vi "Default Settings.vi"(6 "Assembly Type":string, 8 "error in (no error)":errorcluster, 11 "Sensor Dispense in":refnum<class "Sensor Dispense.lvclass">) -> (0 "error out":errorcluster, 3 "Sensor Dispense out":refnum<class "Sensor Dispense.lvclass">)   [LabVIEW 2021, in "Sensor Dispense.lvclass"]
uses:
  Projects/Sensor Dispense.lvclass
  C:/Users/User/Documents/Jessica_Code/Jessica_code_06052024/Gantry-CMU/UCSB-Gantry-HEP-main/Classes/Routine/Dispense/Dispense.lvclass
  Projects/Sensor Dispense.lvclass/Sensor Dispense.ctl
  Dispense.lvclass/Dispense.ctl
  Write Tip Height.vi
  Dispense.lvclass
panel:
  in  "Dispense Type":u16
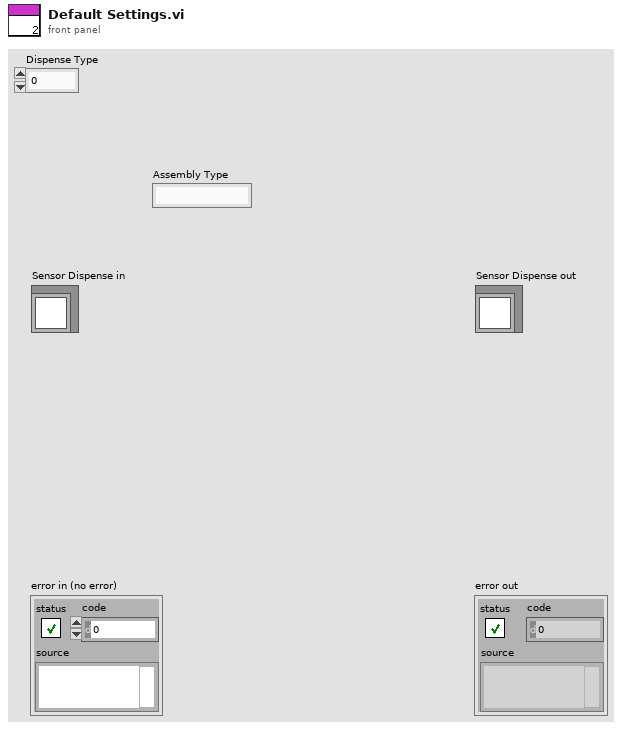
[diagram p1: front panel]
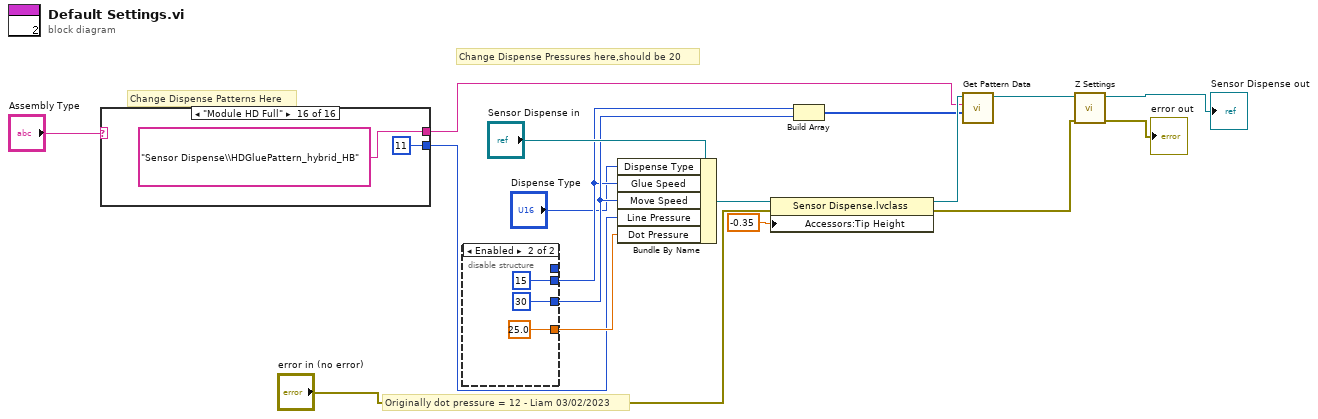
[diagram p0: block diagram]
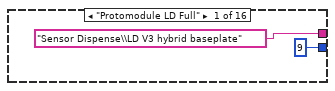
[diagram p2: hidden frame]
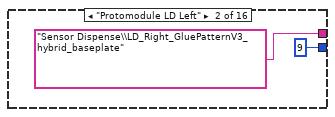
[diagram p3: hidden frame]
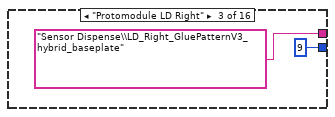
[diagram p4: hidden frame]
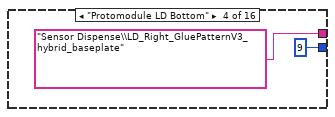
[diagram p5: hidden frame]
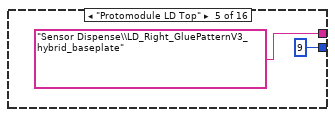
[diagram p6: hidden frame]
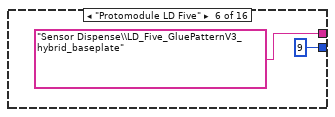
[diagram p7: hidden frame]
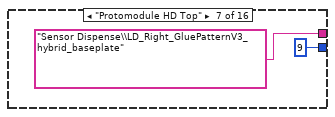
[diagram p8: hidden frame]
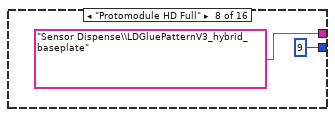
[diagram p9: hidden frame]
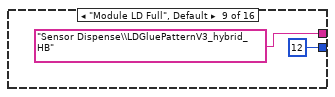
[diagram p10: hidden frame]
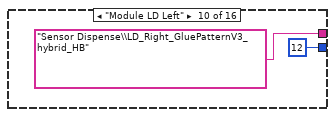
[diagram p11: hidden frame]
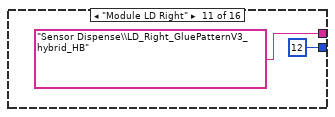
[diagram p12: hidden frame]
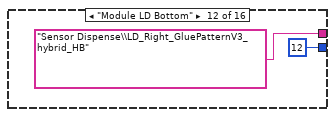
[diagram p13: hidden frame]
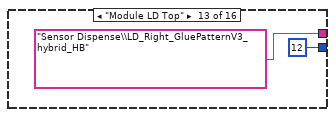
[diagram p14: hidden frame]
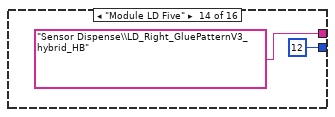
[diagram p15: hidden frame]
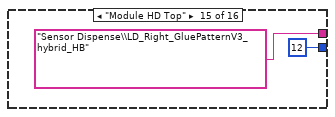
[diagram p16: hidden frame]
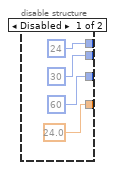
[diagram p17: hidden frame]
diagram:
  # "Change Dispense Patterns Here"
  # "Change Dispense Pressures here,should be 20"
  # "Originally dot pressure = 12 - Liam 03/02/2023"
  n1 = case shown="\"Module HD Full\"" "Assembly Type" {
    tunnel: ["Sensor Dispense\\LD V3 hybrid baseplate" "Sensor Dispense\\LD_Right_GluePatternV3_hybrid_baseplate" "Sensor Dispense\\LD_Right_GluePatternV3_hybrid_baseplate" "Sensor Dispense\\LD_Right_GluePatternV3_hybrid_baseplate" "Sensor Dispense\\LD_Right_GluePatternV3_hybrid_baseplate" "Sensor Dispense\\LD_Five_GluePatternV3_hybrid_baseplate" "Sensor Dispense\\LD_Right_GluePatternV3_hybrid_baseplate" "Sensor Dispense\\LDGluePatternV3_hybrid_baseplate" "Sensor Dispense\\LDGluePatternV3_hybrid_HB" "Sensor Dispense\\LD_Right_GluePatternV3_hybrid_HB" "Sensor Dispense\\LD_Right_GluePatternV3_hybrid_HB" "Sensor Dispense\\LD_Right_GluePatternV3_hybrid_HB" "Sensor Dispense\\LD_Right_GluePatternV3_hybrid_HB" "Sensor Dispense\\LD_Right_GluePatternV3_hybrid_HB" "Sensor Dispense\\LD_Right_GluePatternV3_hybrid_HB" "Sensor Dispense\\HDGluePattern_hybrid_HB"] -> w13
    tunnel: [9 9 9 9 9 9 9 9 12 12 12 12 12 12 12 11] -> w3
    frame "Protomodule LD Full" {
    }
    frame "Protomodule LD Left" {
    }
    frame "Protomodule LD Right" {
    }
    frame "Protomodule LD Bottom" {
    }
    frame "Protomodule LD Top" {
    }
    frame "Protomodule LD Five" {
    }
    frame "Protomodule HD Top" {
    }
    frame "Protomodule HD Full" {
    }
    frame "Module LD Full", Default {
    }
    frame "Module LD Left" {
    }
    frame "Module LD Right" {
    }
    frame "Module LD Bottom" {
    }
    frame "Module LD Top" {
    }
    frame "Module LD Five" {
    }
    frame "Module HD Top" {
    }
    frame "Module HD Full" {
    }
  }
  n2 = disable-structure shown="Enabled" {
    disable-tunnel: [60 30] -> w6
    disable-tunnel: [30 15] -> w5
    disable-tunnel: [24.0 ("Dot Pressure") 25.0 ("Dot Pressure")] -> w4
    disable-tunnel: [24 _] -> _
    frame Disabled {
    }
    frame Enabled {
    }
  }
  n3 = Bundle By Name(cluster="Sensor Dispense in", "Dispense Type"="Dispense Type", "Glue Speed"=w5, "Move Speed"=w6, "Line Pressure"=w3, "Dot Pressure"=w4) -> (w17:refnum<class "Sensor Dispense.lvclass">)
  n4 = property class="Sensor Dispense.lvclass"(reference=w17, error in="error in (no error)", "Accessors:Tip Height"=-0.35) -> (reference out=w14:refnum<class "Sensor Dispense.lvclass">, error out=w8:errorcluster)
  n5 = Build Array(w5, w6) -> (w12:i32[])
  n6 = call "Get Pattern Data.vi"("File Name"=w12, "Folder Name"=w13, "Dispense.lvclass"=w14) -> ("Dispense Out"=w11:refnum<class "Sensor Dispense.lvclass">)  [unwired: 8 in]
  n7 = call-dynamic "Z Settings.vi"("error in (no error)"=w8, "Dispense in"=w11) -> ("error out"=→"error out":errorcluster, "Dispense out"=→"Sensor Dispense out":refnum<class "Sensor Dispense.lvclass">)  [unwired: 8 in]
